vi "XML - Get Groups Content.vi"(8 "error in (no error)":errorcluster, 9 "Rx":T3[](array[typedef]) format="%.0x", 10 "Tx":T3[](array[typedef]) format="%.0x", 11 "Target Ref In":T3 format="%.0x") -> (0 "error IO":errorcluster, 2 "Groups":T1[](array[typedef]) {"Rx Channels"."Data Type" items=["U8", "U16", "U32", "U64", "I8", "I16", "I32", "I64", "SGL", "DBL", "EXT"]; "Tx Channels"."Data Type" items=["U8", "U16", "U32", "U64", "I8", "I16", "I32", "I64", "SGL", "DBL", "EXT"]}, 3 "Target Ref Out":T3 format="%.0x")   [LabVIEW 2016, in "UDP-Custom-Device System Explorer.lvlib"]
doc: "This VI retrieves all different Channels Groups content."
uses:
  UDP-Custom-Device System Explorer.lvlib
  <vilib>/NI Veristand/Custom Device API/Custom Device Item Ref.ctl
  Types/XML/XML - Group.ctl
  Types/XML/XML - Channel.ctl
  <vilib>/NI VeriStand/Custom Device API/Custom Device API.lvlib
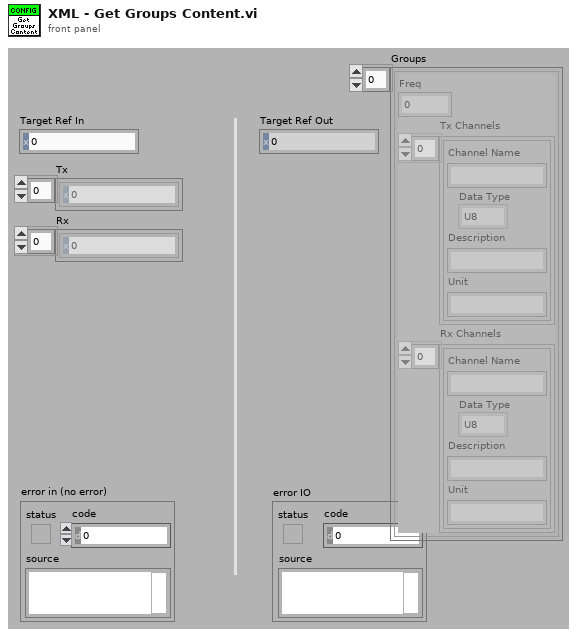
[diagram p1: front panel]
types:
  T1 = typedef "UDP-Custom-Device System Explorer.lvlib/XML - Group.ctl" = cluster{"Freq":i32, "Tx Channels":T2[], "Rx Channels":T2[]}
  T2 = typedef "UDP-Custom-Device System Explorer.lvlib/XML - Channel.ctl" = cluster{"Channel Name":string, "Data Type":u16, "Description":string, "Unit":string}
  T3 = typedef "Custom Device API.lvlib/Custom Device Item Ref.ctl" = u64
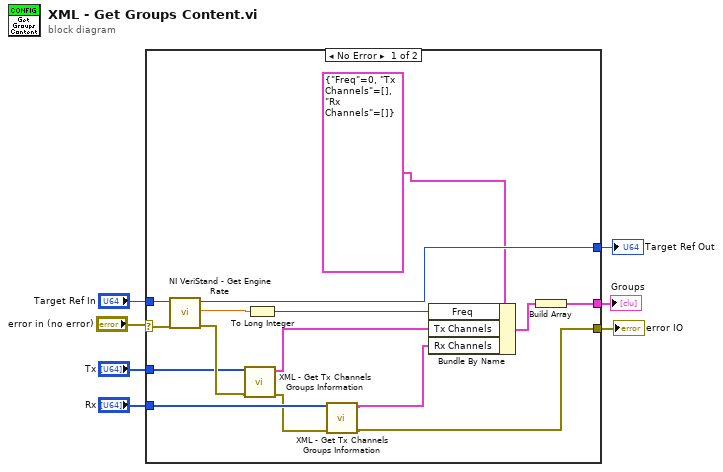
[diagram p0: block diagram]
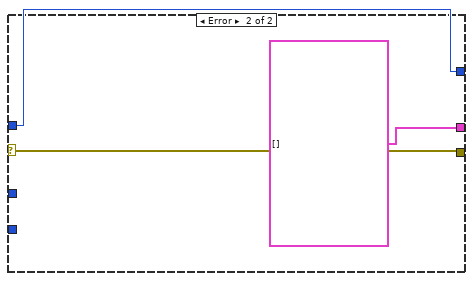
[diagram p2: hidden frame]
diagram:
  n1 = case shown="No Error" "error in (no error)" {
    selector: "error in (no error)" -> [w19 w25]
    tunnel: "Tx" -> [w13 _]
    tunnel: "Rx" -> [w12 _]
    tunnel: "Target Ref In" -> [w22 w24]
    tunnel: [w8 w25] -> w3
    tunnel: [w18 w24] -> w2
    tunnel: [w15 T1[] []] -> w1
    frame No Error {
      n2 = call <vilib>:"NI VeriStand - Get Engine Rate.vi"("error in (no error)"=w19, "Item Ref in"=w22) -> ("error out"=w14:errorcluster, "Rate (Hz)"=w17:dbl, "Item Ref out"=w18:T3)  [unwired: 7 in]
      n3 = call "XML - Get Tx Channels Groups Information.vi"("error in"=w14, "Selected Channel Refs"=w13) -> ("error out"=w11:errorcluster, "Channels"=w10:T2[])  [unwired: 8 in]
      n4 = To Long Integer(number=w17) -> (32bit integer=w21:i32)
      n5 = call "XML - Get Tx Channels Groups Information.vi"("error in"=w11, "Selected Channel Refs"=w12) -> ("error out"=w8:errorcluster, "Channels"=w9:T2[])  [unwired: 8 in]
      n6 = Bundle By Name(cluster=T1 {"Freq"=0, "Tx Channels"=[], "Rx Channels"=[]} ("Group"), "Freq"=w21, "Tx Channels"=w10, "Rx Channels"=w9) -> (w20:T1)
      n7 = Build Array(w20) -> (w15:T1[])
    }
    frame Error {
    }
  }
  "error IO" <- w3
  "Target Ref Out" <- w2
  "Groups" <- w1
